vi "Acquisition Stream Control Core.vi"(0 "SPC":u8=1, 1 "input valid":bool, 2 "request state":T1, 3 "num samples":u64, 4 "initial ignore":u64, 7 "ready for output (T)":bool=TRUE, 8 "reset":bool, 9 "start trigger":bool) -> (10 "cache write index":u8, 11 "ready for start":bool, 12 "cache write enable":bool, 15 "output valid":bool, 16 "actual state":T1, 17 "samples transferred":u64, 19 "acquiring":bool)   [LabVIEW 2018, in "Streaming FPGA.lvlib"]
doc: "<B>General</B>\n\nThis VI controls the signal acquisition data flow with a state machine controller. This enables the control and monitoring of finite and continuous streams of data between nodes using 4-wire handshaking. This VI provides control signals for the data transfer, but it does not handle the data transfer itself.\n\n<B>Signals</B>\n\nThe stream is controlled by the <B>request state</B>, <B>num samples</B>, <B>initial ignore</B> and <B>start trigger</B> inputs. The stream is monitored by the <B>actual state</B>, <B>ready for start</B>, <B>samples transferred</B> and <B>acquiring</B> outputs.\n\nThe upstream node can provide data by setting the <B>input valid</B> input to true. The data provided by the upstream node is accepted if the <B>input valid</B> input is true.\n\nThe <B>output valid</B> output is set to true when data is available. The downstream node should set the <B>ready for output</B> input to true when it is ready for data. If the <B>ready for output</B> input is true and the <B>output valid</B> output is also true, then the downstream node should accept the data provided. If the <B>ready for output</B> input is false or if the <B>output valid</B> output is false, then the downstream should ignore the data provided.\n\nNote that this VI doesn't have a \"ready for input\" output. The data provided by the upstream node is always accepted, but if an acquisition is in progress and the downstream node is not able to accept the data provided by the upstream node, then the acquisition aborts.\n\n<B>Data movement control signals</B>\n\nThe <B>SPC</B> input should be set to the number of samples per clock cycle used by the upstream and downstream nodes. This VI assumes that the caller VI has a <B>data in</B> data input and a <B>data out</B> data output which are arrays of <B>SPC</B> number of samples. This VI also assumes that the caller implements a cache register which is an array of <B>SPC</B>-1 number of samples and an output register which is an array of <B>SPC</B> number of samples. In each cycle the caller VI should update these registers and the <B>data out</B> data output in the following way:\n- Take the cache register output array and resize it to 2*<B>SPC</B>-1 number of elements. Denote the resulting array C1.\n- Replace a subset of the C1 array starting from the <B>cache write index</B> index using the <B>data in</B> data input as the new subarray (the <B>cache write index</B> output is always between 0 and <B>SPC</B>-1).\n- Write the output register using the first <B>SPC</B> number of elements from the C1 array.\n- If the <B>cache write enable</B> output is true, then write the cache register using the last <B>SPC</B>-1 number of elements from the C1 array. If the <B>cache write enable</B> output is false, then do not write the cache register.\n- Write the <B>data out</B> data output by the output register output.\n\n<B>Detailed Operation</B>\n\nIf an acquisition is in progress, then the samples provided on the data input are returned on the data output. If no acquisition is in progress then the samples provided on the data input are ignored.\n\nThere are two signal acquisition modes: finite or continuous mode. Each time a signal acquisition is started the controller ignores <B>initial ignore</B> number of input samples, then transfers <B>num samples</B> samples (in case of finite mode) or an unspecified number of samples (in case of continuous mode) from the data input to the data output. A finite signal acquisition can be started by transitioning the state machine from the Idle state to the Finite Transfer state. A continuous signal acquisition can be started by transitioning the state machine from the Idle state to the Continuous state. Transitioning from the Idle state to the Finite Transfer or Continuous state does not start the signal acquisition immediately, when transitioning into these states the state machine always waits for a start trigger before starting the acquisition. The state machine sets the <B>ready for start</B> output to true when it is waiting for a start trigger in the next cycle (otherwise this output is false), the start trigger can be provided on the <B>start trigger</B> input by setting this input to true. The acquisition starts in the cycle when the <B>start trigger</B> input is true and the <B>ready for start</B> output was true in the previous cycle. The data provided on the data input in this cycle is the first data input that is part of the acquisition. The start of the acquisition is also signaled by the <B>acquiring</B> output becoming true. This output is set to false when the acquisition ends. Note that this VI assumes that the signal acquisition should be continuous: during the signal acquisition if the <B>ready for output</B> input is false while data is available on the data output, the state machine aborts the signal acquisition and enters the Error state.\n\n<B>samples transferred</B> is updated with the number of upstream node provided samples accepted by the downstream node in the current cycle, that is, this counter does not include the number of initial samples ignored during the acquisition.\n\nIn finite mode the state machine enters the Done state once the signal acquisition is finished. In the Done state the samples transferred continues to be reported until the user requests that the state machine return to Idle. A signal acquisition can be aborted by entering the Cancel state. When entering the Cancel state, the state machine transitions to the Not Ready state, then it can transition into the Idle state.\n\nIn order to reset this VI set the <B>request state</B> input to Idle, set the <B>reset</B> input to true, wait until the <B>actual state</B> output indicates Idle, then set the <B>reset</B> input to false.\n\n<b>States</b>\n\nThere are seven potential states for a stream defined by the Stream State.ctl typedef. All commanded states should be monitored from the controlling loop if it is important to ensure that the state is actually entered. The <B>request state</B> commands the stream into a state, and <B>actual state</B> reflects the current actual state.\n\nIdle - when the stream is ready to enter into an active state, it is in the Idle state. While it can be commanded directly to Idle from any state, it is advisable to do so with caution as samples abandoned in transfers may still need to be manually cleared out. It is generally safe to go directly from Done to Idle, and it is generally safe to request a transition from Not Ready to Idle. Other states may require further clean-up such as stopping/starting FIFOs or resetting other code under the command of the stream. Consider using Cancel instead (such as through the \"Stop Stream.vi\" in the host environment). While in Idle, <B>samples transferred</B> is reset to 0.\n\nFinite Transfer - Execute a transfer for the requested number of samples. Upon an orderly completion, this VI will automatically enter the Done state. If a stream overflows because the <B>ready for output</B> input is false while data is available on the data output, then the state machine enters the Error state.\n\nContinuous - Execute a transfer indefinitely. This state operates identically to the Finite Transfer state, but without regard to the <B>num samples</B> input.\n\nDone - In an orderly termination of a finite stream, the stream should end up here. At this point, <B>samples transferred</B> accurately reflects the terminal state of the transfer. The Done state should be exited by requesting Idle. Further active transfer modes (Finite or Continuous) will be ignored. This allows the host to distinguish between streams that are prematurely terminated (thus potentially requiring a flush of abandoned data) and ones that completed naturally.\n\nError - If the stream detects an unplanned interruption of the data, it enters the Error state. The only way to exit the Error state is to command the Acquisition Stream Control to Idle or Not Ready. When commanded to Idle or Not Ready, the Acquisition Stream Control advances first to Not Ready.\n\nNot Ready - In this state, the Acquisition Stream Control remains in the Not Ready state until it is commanded to Idle. This prevents starting a transfer in an obviously invalid state, and allows host control to wait until the not ready state is removed (such as by clearing out a FIFO under the streaming API's control).\n\nCancel - This state is indistinguishable from Error, but allows the controlling VI to know what condition caused the transfer to terminate."
uses:
  Streaming FPGA.lvlib
  <instrlib>/_niInstr/Streaming/v1/Common/Stream State.ctl
  <instrlib>/_niInstr/Streaming/v1/Common/niInstr Streaming v1 Common.lvlib
  <instrlib>/_niInstr/Basic Elements/v1/FPGA/niInstr Basic Elements v1 FPGA.lvlib
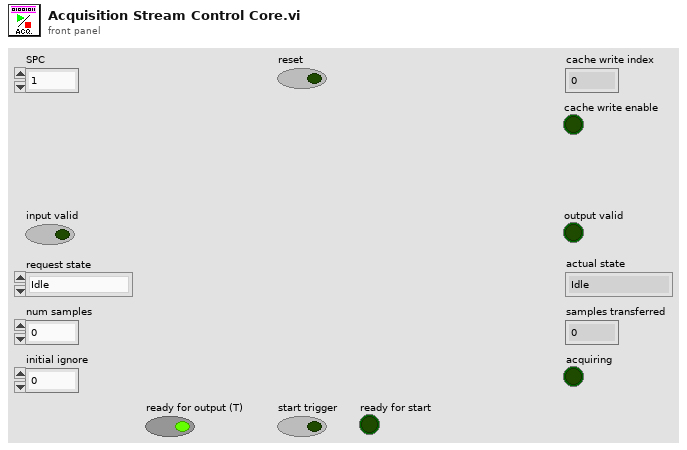
[diagram p1: front panel]
types:
  T1 = typedef "niInstr Streaming v1 Common.lvlib/Stream State.ctl" = enum8{"Idle", "Finite Transfer", "Continuous", "Done", "Error", "Not Ready", "Cancel"}
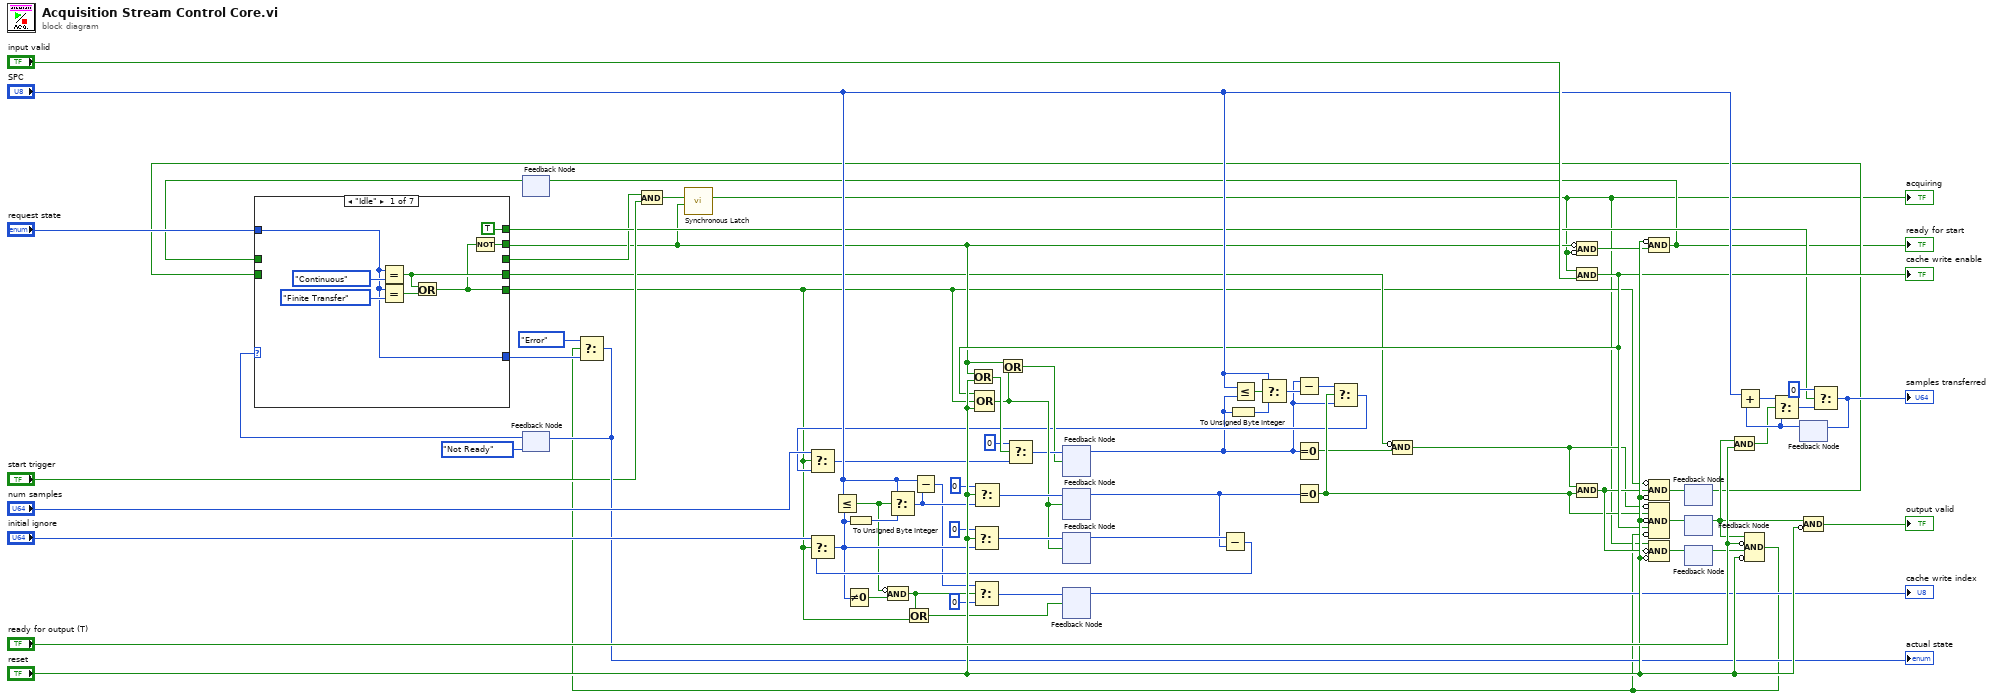
[diagram p0: block diagram]
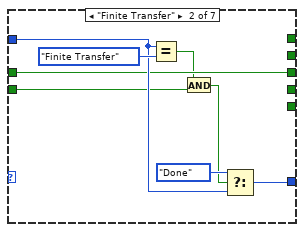
[diagram p2: hidden frame]
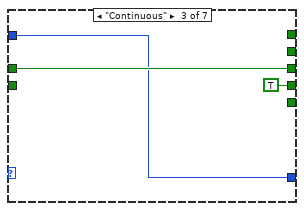
[diagram p3: hidden frame]
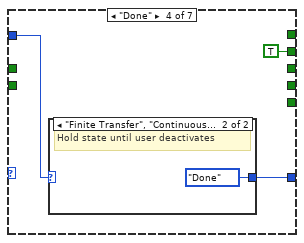
[diagram p4: hidden frame]
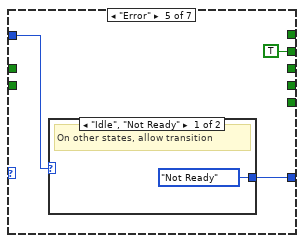
[diagram p6: hidden frame]
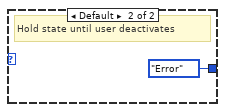
[diagram p7: hidden frame]
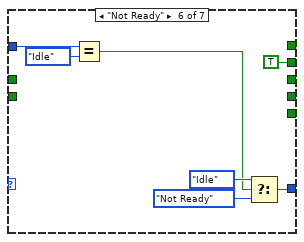
[diagram p8: hidden frame]
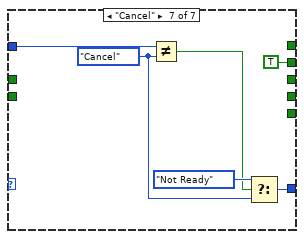
[diagram p9: hidden frame]
diagram:
  n1 = feedback #1() -> (w56:bool)  [unwired: 1 in]
  n2 = feedback #2(Stream_State."Not Ready" ("request state")) -> (w48:T1)
  n3 = feedback #3() -> (w11:u64)  [unwired: 1 in]
  n4 = feedback #4() -> (w16:u8)  [unwired: 1 in]
  n5 = feedback #5() -> (w35:u64)  [unwired: 1 in]
  n6 = feedback #6() -> (→"cache write index":u8)  [unwired: 1 in]
  n7 = Subtract(x=w35, y=w16) -> (x-y=w27:u64)
  n8 = To Unsigned Byte Integer(number=w11) -> (unsigned 8bit integer=w37:u8)
  n9 = Less Or Equal?(x="SPC", y=w11) -> (x <= y?=w58:bool)
  n10 = Select(t="SPC", s=w58, f=w37) -> (s? t:f=w15:u8)
  n11 = Subtract(x=w11, y=w15) -> (x-y=w13:u64)
  n12 = Equal To 0?(x=w11) -> (x = 0?=w10:bool)
  n13 = Equal To 0?(x=w16) -> (x = 0?=w14:bool)
  n14 = Select(t=w13, s=w14, f=w11) -> (s? t:f=w12:u64)
  n15 = feedback #7() -> (w6:bool)  [unwired: 1 in]
  n16 = case shown="\"Idle\"" w48 {
    tunnel: "request state" -> [w76 w87 w89 w94 w99 w108 w114]
    tunnel: [w76 w85 w89 w93 w98 w106 w112] -> w45
    tunnel: [w74 _ _ _ _ _ _] -> w4
    tunnel: [w77 _ TRUE _ _ _ _] -> w9
    tunnel: [TRUE _ _ _ _ _ _] -> w49
    tunnel: w6 -> [_ w83 _ _ _ _ _]
    tunnel: w56 -> [_ w82 w91 _ _ _ _]
    tunnel: [_ w82 w91 _ _ _ _] -> w42
    tunnel: [w73 _ _ TRUE TRUE TRUE TRUE] -> w26
    frame "Idle" {
      n17 = Equal?(x=w76, y=Stream_State."Continuous") -> (x = y?=w77:bool)
      n18 = Equal?(x=w76, y=Stream_State."Finite Transfer") -> (x = y?=w78:bool)
      n19 = Or(x=w77, y=w78) -> (x .or. y?=w74:bool)
      n20 = Not(x=w74) -> (.not. x?=w73:bool)
    }
    frame "Finite Transfer" {
      n21 = Equal?(x=w87, y=Stream_State."Finite Transfer") -> (x = y?=w81:bool)
      n22 = And(x=w81, y=w83) -> (x .and. y?=w84:bool)
      n23 = Select(t=Stream_State."Done", s=w84, f=w87) -> (s? t:f=w85:T1)
    }
    frame "Continuous" {
    }
    frame "Done" {
      n24 = case shown="\"Finite Transfer\", \"Continuous\"" w94 {
        selector: w94 -> [w95 _]
        tunnel: [w95 Stream_State."Done" ("request state")] -> w93
        frame Default {
          # "On other states, allow transition"
        }
        frame "Finite Transfer", "Continuous" {
          # "Hold state until user deactivates"
        }
      }
    }
    frame "Error" {
      n25 = case shown="\"Idle\", \"Not Ready\"" w99 {
        tunnel: [Stream_State."Not Ready" ("t") Stream_State."Error" ("request state")] -> w98
        frame "Idle", "Not Ready" {
          # "On other states, allow transition"
        }
        frame Default {
          # "Hold state until user deactivates"
        }
      }
    }
    frame "Not Ready" {
      n26 = Equal?(x=w108, y=Stream_State."Idle") -> (x = y?=w102:bool)
      n27 = Select(t=Stream_State."Idle" ("y"), s=w102, f=Stream_State."Not Ready") -> (s? t:f=w106:T1)
    }
    frame "Cancel" {
      w113 = Stream_State."Cancel" ("y")
      n28 = Not Equal?(x=w114, y=w113) -> (x != y?=w109:bool)
      n29 = Select(t=Stream_State."Not Ready", s=w109, f=w113) -> (s? t:f=w112:T1)
    }
  }
  n30 = And(x=w42, y="start trigger") -> (x .and. y?=w57:bool)
  n31 = call <instrlib>:"Synchronous Latch.vi"("clear"=w26, "set"=w57) -> ("out"=w1:bool)  [unwired: 9 in]
  "acquiring" <- w1
  n32 = Select(t="num samples", s=w4, f=w12) -> (s? t:f=w30:u64)
  n33 = Select(t="initial ignore", s=w4, f=w27) -> (s? t:f=w24:u64)
  n34 = Less Or Equal?(x="SPC", y=w24) -> (x <= y?=w22:bool)
  n35 = Not Equal To 0?(x=w24) -> (x != 0?=w23:bool)
  n36 = To Unsigned Byte Integer(number=w24) -> (unsigned 8bit integer=w34:u8)
  n37 = Compound Arithmetic op=AND(invert w22, w23) -> (w19:bool)
  n38 = Select(t="SPC", s=w22, f=w34) -> (s? t:f=w25:u8)
  n39 = Or(x=w19, y=w4) -> (x .or. y?=w17:bool)
  n40 = Subtract(x="SPC", y=w25) -> (x-y=w21:u8)
  n41 = Or(x=w26, y="reset") -> (x .or. y?=w59:bool)
  n42 = Select(t=u64 0, s="reset", f=w24) -> (s? t:f=w39:u64)
  n43 = Select(t=w21, s=w19, f=u8 0) -> (s? t:f=w18:u8)
  n44 = Select(t=u8 0, s="reset", f=w25) -> (s? t:f=w33:u8)
  n45 = Select(t=u64 0, s=w59, f=w30) -> (s? t:f=w29:u64)
  n46 = feedback-in #6(w18, w17) -> ()
  n47 = Compound Arithmetic op=AND(invert w9, w10) -> (w8:bool)
  n48 = And(x=w1, y="input valid") -> (x .and. y?=w61:bool)
  "cache write enable" <- w61
  n49 = Compound Arithmetic op=OR(w61, w4, "reset") -> (w31:bool)
  n50 = Or(x=w26, y=w31) -> (x .or. y?=w28:bool)
  n51 = feedback-in #3(w29, w28) -> ()
  n52 = feedback-in #4(w33, w31) -> ()
  n53 = feedback-in #5(w39, w31) -> ()
  n54 = Compound Arithmetic op=AND(invert w26, invert w1) -> (w41:bool)
  n55 = Compound Arithmetic op=AND(w8, w14) -> (w47:bool)
  n56 = Compound Arithmetic op=AND(invert "reset", w41) -> (w2:bool)
  "ready for start" <- w2
  n57 = feedback-in #1(w2) -> ()
  n58 = Compound Arithmetic op=AND(invert w4, w47, invert "reset") -> (w5:bool)
  n59 = Compound Arithmetic op=AND(w1, invert w47, invert "reset") -> (w46:bool)
  n60 = feedback-in #7(w5) -> ()
  n61 = feedback #8() -> (w36:bool)  [unwired: 1 in]
  n62 = feedback #9() -> (w43:bool)  [unwired: 1 in]
  n63 = feedback-in #9(w46) -> ()
  n64 = And(x=w36, y="ready for output (T)") -> (x .and. y?=w7:bool)
  n65 = Compound Arithmetic op=AND(w36, invert "ready for output (T)", w43, invert "reset") -> (w3:bool)
  n66 = Select(t=Stream_State."Error", s=w3, f=w45) -> (s? t:f=w64:T1)
  "actual state" <- w64
  n67 = feedback-in #2(w64) -> ()
  n68 = Compound Arithmetic op=AND(invert w8, w14, invert "reset", w61, invert w3) -> (w54:bool)
  n69 = feedback-in #8(w54) -> ()
  n70 = feedback #10() -> (w52:u64)  [unwired: 1 in]
  n71 = Add(x="SPC", y=w52) -> (x+y=w53:u64)
  n72 = Select(t=w53, s=w7, f=w52) -> (s? t:f=w51:u64)
  n73 = Compound Arithmetic op=AND(w36, invert "reset") -> (→"output valid":bool)
  n74 = Select(t=u64 0, s=w49, f=w51) -> (s? t:f=w66:u64)
  "samples transferred" <- w66
  n75 = feedback-in #10(w66) -> ()
